vi "Untitled 3.vi"() -> ()   [LabVIEW 2018]
panel:
  out "Array 2":bool[][](array[boolean])
  out "Array":bool[][](array[boolean])
  out "output array":bool[](array[boolean])
  out "x+y":u8
  in  "Numeric":u8
  # "M"
  # "L"
  # "0"
  # "1"
  # "2"
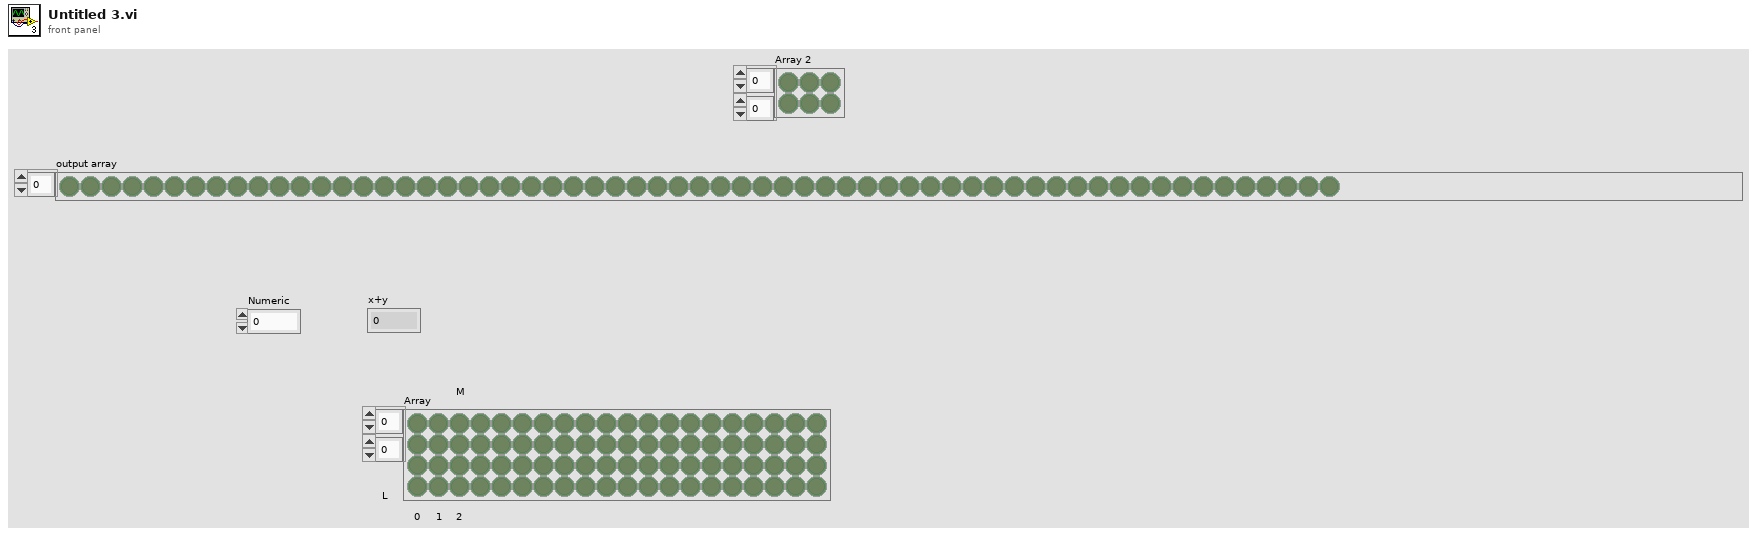
[diagram p1: front panel]
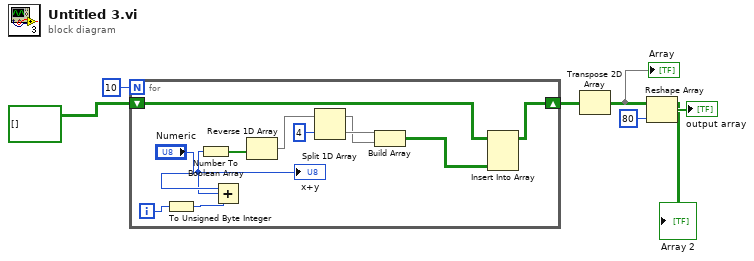
[diagram p0: block diagram]
diagram:
  n1 = for {
    N: 10 -> [_]
    shift-right: [w7] -> w2
    shift-left: bool[][] [] -> [w8]
    i -> [w11]
    n2 = To Unsigned Byte Integer(number=w11) -> (unsigned 8bit integer=w10:u8)
    n3 = Add(x="Numeric", y=w10) -> (x+y=w12:u8)
    "x+y" <- w12
    n4 = Number To Boolean Array(number=w12) -> (Boolean array=w17:bool[])
    n5 = Reverse 1D Array(array=w17) -> (reversed array=w16:bool[])
    n6 = Split 1D Array(array=w16, index=4) -> (first subarray=w14:bool[], second subarray=w15:bool[])
    n7 = Build Array(w15, w14) -> (w9:bool[][])
    n8 = Insert Into Array(array=w8, new element=w9) -> (w7:bool[][])  [unwired: 2 in]
  }
  "Array 2" <- w2
  n9 = Transpose 2D Array(2D array=w2) -> (transposed array=w1:bool[][])
  "Array" <- w1
  n10 = Reshape Array(w1, 80 ("dimension size")) -> (→"output array":bool[])
